vi "LVCAM Msg Drop.vi"(10 "Remaining Elements":refnum<class "Msg.lvclass">[](array[class]), 11 "LVCAM Msg Drop in":refnum<class "LVCAM Msg Drop.lvclass">) -> (3 "LVCAM Msg Drop out":refnum<class "LVCAM Msg Drop.lvclass">)   [LabVIEW 2021, in "LVCAM.lvlib" / "LVCAM Msg Drop.lvclass"]
uses:
  LVCAM Msg Drop.lvclass
  Msg/Msg.lvclass
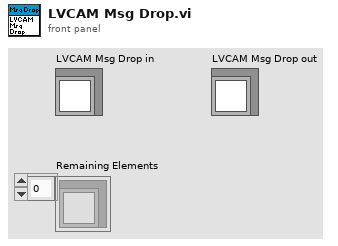
[diagram p1: front panel]
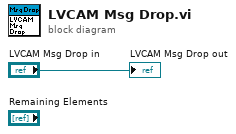
[diagram p0: block diagram]
diagram:
  "LVCAM Msg Drop out" <- "LVCAM Msg Drop in"
